vi "Array1D_Operations.vi"() -> ()   [LabVIEW 2019]
uses:
  97f7c315-10c0-4470-b7b1-4ed5093533e2.vi
  ddde8835-4f6d-40b5-a6f5-9b8c625cb98e.vi
  d9a6163d-5506-418f-b037-04e918bcd0f3.vi
panel:
  out "array A with decremented value at A[0] by 1":u8[](array[numeric])
  out "array A with incremented value at A[3] by 1":u8[](array[numeric])
  out "reversed array":u8[](array[numeric])
  out "shuffled array":u8[](array[numeric])
  out "sorted array(decremented order)":u8[](array[numeric])
  out "min index(A)":i32
  out "min value(A)":u8
  out "max index(A)":i32
  out "max value(A)":u8
  out "array with subset B deleted":u8[](array[numeric])
  in  "B (Array)":u8[](array[numeric])=[8, 7, 6, 5]
  out "Inserting Array B into A":u8[](array[numeric])
  out "Changed A[0]=4 to A[0]=5":u8[](array[numeric])
  out "2nd Element in A":u8
  out "size of A":i32
  in  "A (Array)":u8[](array[numeric])=[4, 3, 2, 1]
  # "Output"
  # "Input"
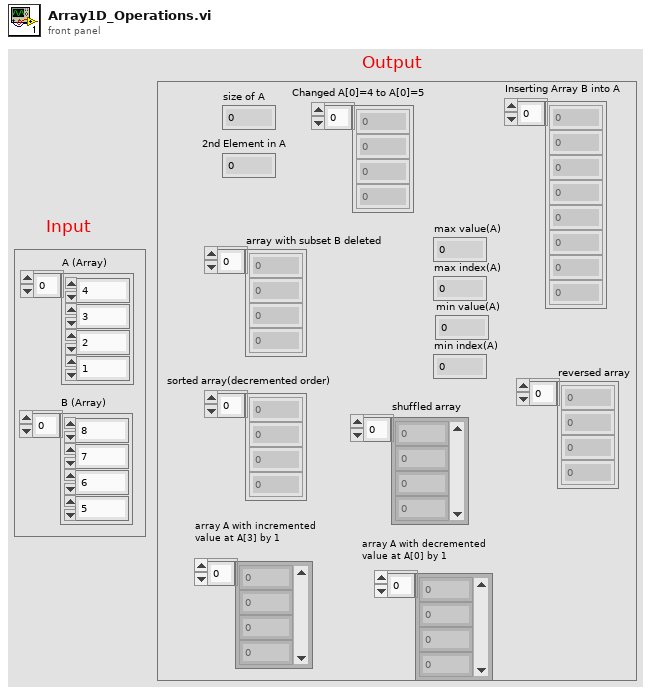
[diagram p1: front panel]
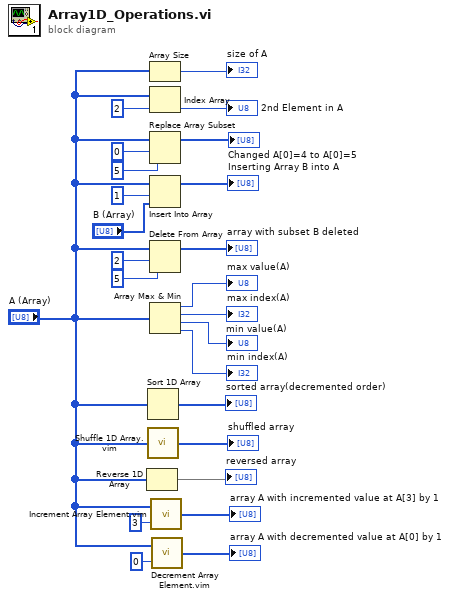
[diagram p0: block diagram]
diagram:
  n1 = Reverse 1D Array(array="A (Array)") -> (reversed array=→"reversed array":u8[])
  n2 = Sort 1D Array(array="A (Array)") -> (sorted array=→"sorted array(decremented order)":u8[])
  n3 = call "Shuffle 1D Array.vim"("array"="A (Array)") -> ("shuffled array"=→"shuffled array":u8[])  [unwired: 4 in]
  n4 = Array Size(array="A (Array)") -> (size(s)=→"size of A":i32)
  n5 = Index Array(array="A (Array)", index=2) -> (element=→"2nd Element in A":u8)
  n6 = Replace Array Subset(array="A (Array)", new element=u8 5 ("new element/subarray"), index=0) -> (→"Changed A[0]=4 to A[0]=5":u8[])
  n7 = Insert Into Array(array="A (Array)", index=1, new element="B (Array)") -> (→"Inserting Array B into A":u8[])
  n8 = Delete From Array(array="A (Array)", length=2, index=5) -> (array with subset deleted=→"array with subset B deleted":u8[])  [unwired: 1 out]
  n9 = Array Max & Min(array="A (Array)") -> (max value=→"max value(A)":u8, max index (indices)=→"max index(A)":i32, min value=→"min value(A)":u8, min index (indices)=→"min index(A)":i32)
  n10 = call "Increment Array Element.vim"("index"=3, "array in"="A (Array)") -> ("array out"=→"array A with incremented value at A[3] by 1":u8[])
  n11 = call "Decrement Array Element.vim"("index"=0, "array in"="A (Array)") -> ("array out"=→"array A with decremented value at A[0] by 1":u8[])
